vi "read_attributes.vi"(8 "error in (no error)":errorcluster, 11 "LarsCV in":refnum<class "LarsCV.lvclass">) -> (0 "error out":errorcluster, 2 "attributes":T1, 3 "LarsCV out":refnum<class "LarsCV.lvclass">)   [LabVIEW 2020, in "LarsCV.lvclass"]
uses:
  LarsCV.lvclass
  Controls/lars_cv_attributes.ctl
  LarsCV.lvclass/LarsCV.ctl
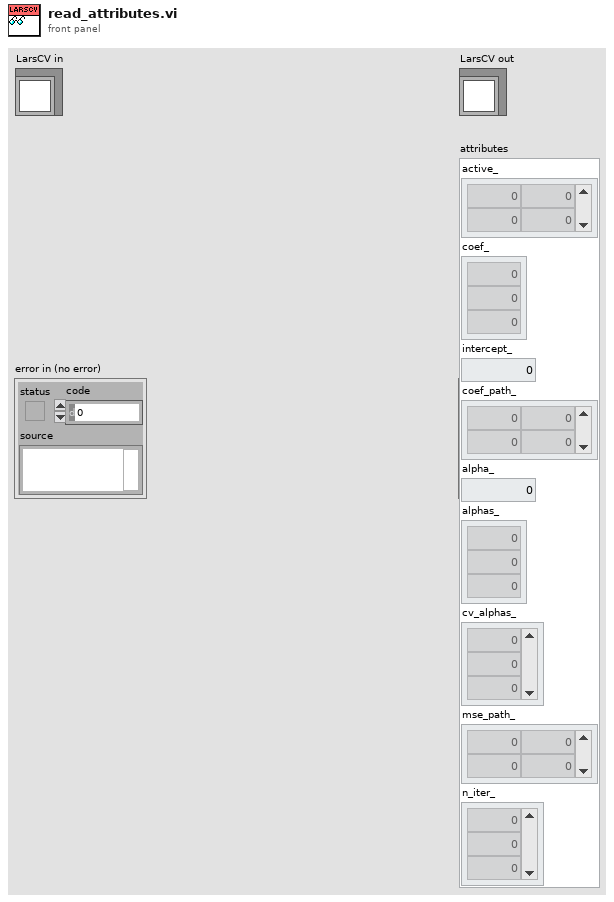
[diagram p1: front panel]
types:
  T1 = typedef "lars_cv_attributes.ctl" = cluster{"active_":dbl[][], "coef_":dbl[], "intercept_":dbl, "coef_path_":dbl[][][], "alpha_":dbl, "alphas_":dbl[], "cv_alphas_":dbl[], "mse_path_":dbl[][], "n_iter_":dbl[]}
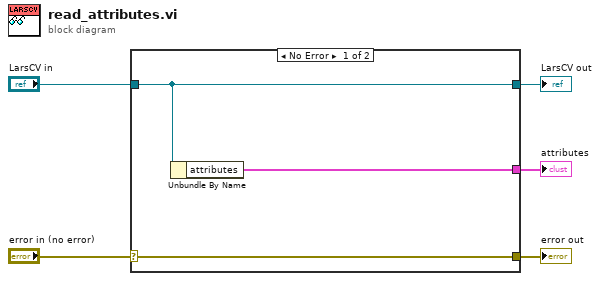
[diagram p0: block diagram]
diagram:
  n1 = case shown="No Error" "error in (no error)" {
    selector: "error in (no error)" -> [w8 w9]
    tunnel: [w8 w9] -> w4
    tunnel: [w7 w10] -> w2
    tunnel: "LarsCV in" -> [w7 w10]
    tunnel: [w6 _] -> w1
    frame No Error {
      n2 = Unbundle By Name(w7) -> ("attributes"=w6:T1)
    }
    frame Error {
    }
  }
  "error out" <- w4
  "LarsCV out" <- w2
  "attributes" <- w1
